vi "z-score.vi"(0 "Array":dbl[](array[numeric])) -> (1 "Mean":dbl, 2 "Standard Deviation":dbl, 3 "Z-Score":dbl[](array[numeric]))   [LabVIEW 2012]
uses:
  <vilib>/Analysis/NI_AALBase.lvlib
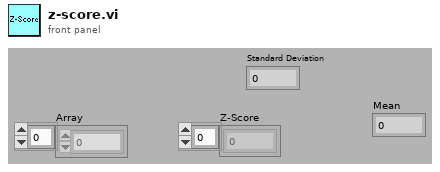
[diagram p1: front panel]
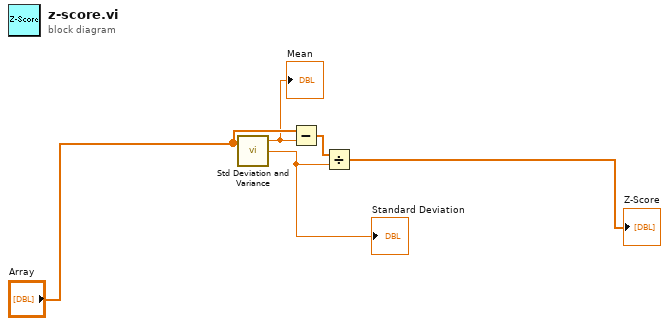
[diagram p0: block diagram]
diagram:
  n1 = call <vilib>:"Std Deviation and Variance.vi"("X"="Array") -> ("mean"=w2:dbl, "standard deviation"=w1:dbl)  [unwired: 1 in, 1 out]
  "Standard Deviation" <- w1
  "Mean" <- w2
  n2 = Subtract(x="Array", y=w2) -> (x-y=w4:dbl[])
  n3 = Divide(x=w4, y=w1) -> (x/y=→"Z-Score":dbl[])
